vi "Clean List of Properties Selection by Type.vi"(11 "Data Cluster in":T1) -> (0 "List of Tags":string[](array[string]), 3 "output cluster":T1)   [LabVIEW 2020, in "Control Property Tree.lvlib"]
uses:
  Control Property Tree.lvlib
  Module Data--cluster.ctl
  Ctrl Properties Map Data.ctl
  Property array.ctl
  Selected Ctrls - List of Controls.ctl
  Selected Ctrls - List of Properties.ctl
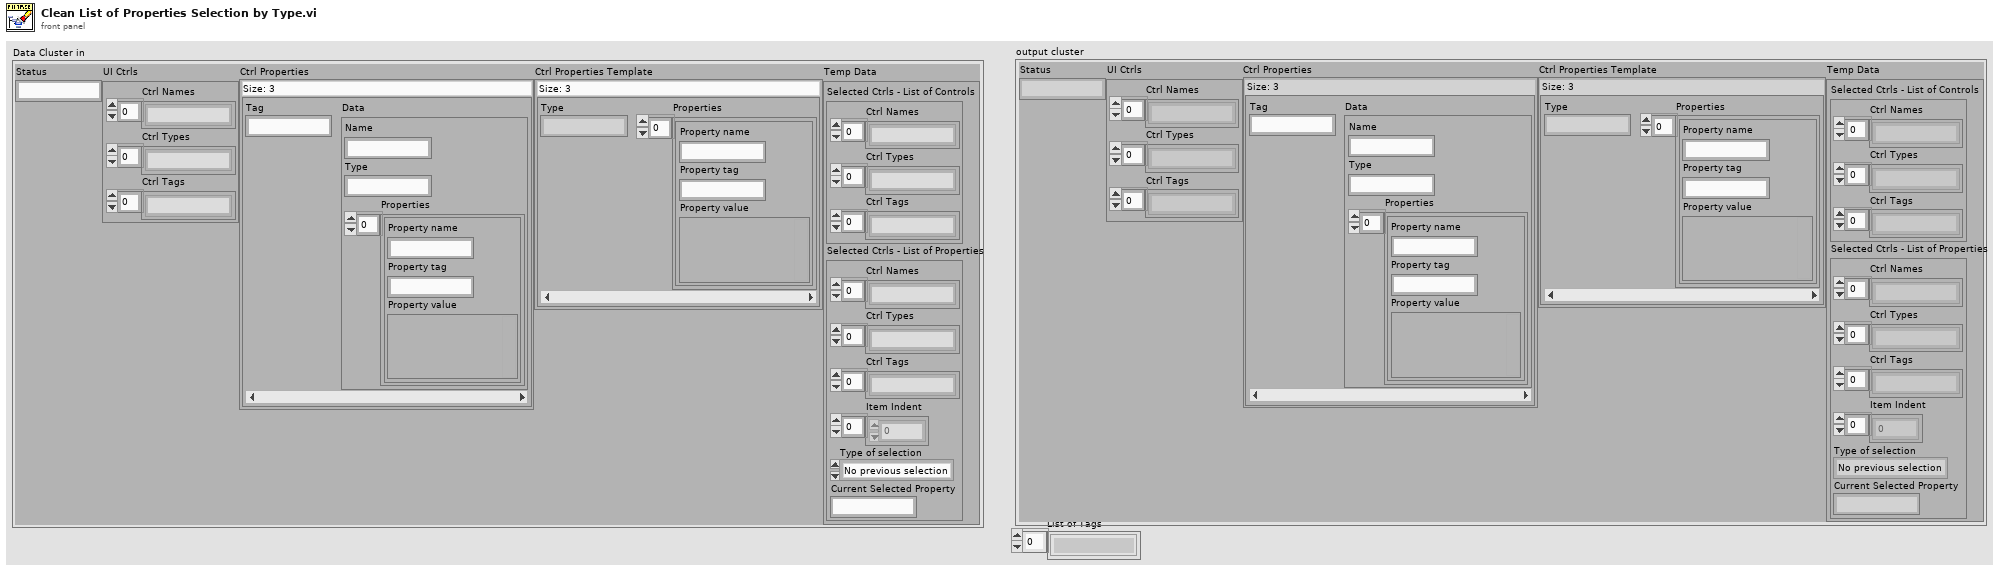
[diagram p1: front panel]
types:
  T1 = typedef "Control Property Tree.lvlib/Module Data--cluster.ctl" = cluster{"Status":string, "UI Ctrls":cluster{"Ctrl Names":string[], "Ctrl Types":string[], "Ctrl Tags":string[]}, "Ctrl Properties":map{string, T2}, "Ctrl Properties Template":map{string, T3}, "Temp Data":cluster{"Selected Ctrls - List of Controls":T4, "Selected Ctrls - List of Properties":T5}}
  T2 = typedef "Control Property Tree.lvlib/Ctrl Properties Map Data.ctl" = cluster{"Name":string, "Type":string, "Properties":T3}
  T3 = typedef "Control Property Tree.lvlib/Property array.ctl" = cluster{"Property name":string, "Property tag":string, "Property value":variant}[]
  T4 = typedef "Control Property Tree.lvlib/Selected Ctrls - List of Controls.ctl" = cluster{"Ctrl Names":string[], "Ctrl Types":string[], "Ctrl Tags":string[]}
  T5 = typedef "Control Property Tree.lvlib/Selected Ctrls - List of Properties.ctl" = cluster{"Ctrl Names":string[], "Ctrl Types":string[], "Ctrl Tags":string[], "Item Indent":i32[], "Type of selection":enum16{"No previous selection", "Control selected", "Property selected"}, "Current Selected Property":string}
  T6 = enum16{"No previous selection", "Control selected", "Property selected"}
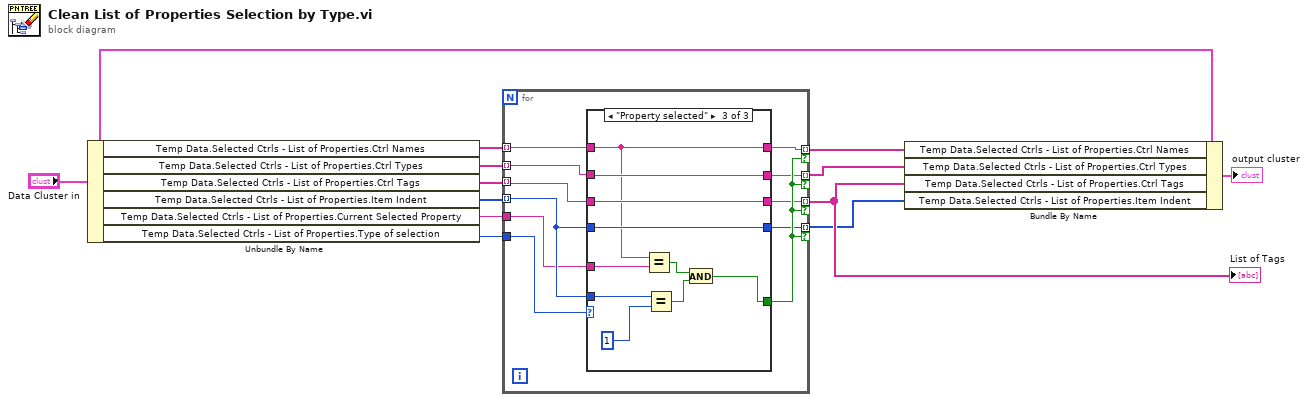
[diagram p0: block diagram]
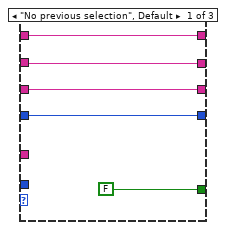
[diagram p2: hidden frame]
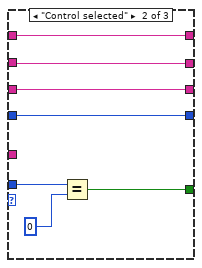
[diagram p3: hidden frame]
diagram:
  n1 = Unbundle By Name("Data Cluster in") -> ("Temp Data.Selected Ctrls - List of Properties.Ctrl Names"=w6:string[], "Temp Data.Selected Ctrls - List of Properties.Ctrl Types"=w5:string[], "Temp Data.Selected Ctrls - List of Properties.Ctrl Tags"=w4:string[], "Temp Data.Selected Ctrls - List of Properties.Item Indent"=w3:i32[], "Temp Data.Selected Ctrls - List of Properties.Current Selected Property"=w1:string, "Temp Data.Selected Ctrls - List of Properties.Type of selection"=w2:T6)
  n2 = for {
    tunnel: w5 -> [w19] mode=indexing
    tunnel: w6 -> [w20] mode=indexing
    tunnel: w4 -> [w16] mode=indexing
    tunnel: w3 -> [w14] mode=indexing
    tunnel: w2 -> [w23]
    tunnel: [w21] -> w12 mode=indexing if=w22
    tunnel: [w18] -> w11 mode=indexing if=w22
    tunnel: [w17] -> w10 mode=indexing if=w22
    tunnel: [w15] -> w9 mode=indexing if=w22
    tunnel: w1 -> [w13]
    n3 = case shown="\"Property selected\"" w23 {
      tunnel: w14 -> [_ w34 w44]
      tunnel: [FALSE w33 w36] -> w22
      tunnel: [w27 w32 w39] -> w21
      tunnel: w20 -> [w27 w32 w39]
      tunnel: w19 -> [w26 w31 w43]
      tunnel: [w26 w31 w43] -> w18
      tunnel: [w25 w30 w42] -> w17
      tunnel: w16 -> [w25 w30 w42]
      tunnel: [w24 w29 w41] -> w15
      tunnel: w14 -> [w24 w29 w41]
      tunnel: w13 -> [_ _ w40]
      frame "No previous selection", Default {
      }
      frame "Control selected" {
        n4 = Equal?(x=w34, y=0) -> (x = y?=w33:bool)
      }
      frame "Property selected" {
        n5 = Equal?(x=w39, y=w40) -> (x = y?=w38:bool)
        n6 = Equal?(x=w44, y=1) -> (x = y?=w37:bool)
        n7 = And(x=w38, y=w37) -> (x .and. y?=w36:bool)
      }
    }
  }
  "List of Tags" <- w10
  n8 = Bundle By Name(cluster="Data Cluster in", "Temp Data.Selected Ctrls - List of Properties.Ctrl Names"=w12, "Temp Data.Selected Ctrls - List of Properties.Ctrl Types"=w11, "Temp Data.Selected Ctrls - List of Properties.Ctrl Tags"=w10, "Temp Data.Selected Ctrls - List of Properties.Item Indent"=w9) -> (→"output cluster":T1)
